vi "GetPktLoss.vi"(8 "error in (no error)":errorcluster, 11 "NetworkPluginNone":refnum<class "NetworkPluginNone.lvclass">) -> (0 "error out":errorcluster, 3 "NetworkPluginNone":refnum<class "NetworkPluginNone.lvclass">)   [LabVIEW 2014, in "NetworkImpairmentPlugins.lvlib" / "NetworkPluginNone.lvclass"]
uses:
  NetworkPluginNone.lvclass
  NetworkImpairmentPluginBase_class/Accessors/Read TimeArray.vi
  NetworkImpairmentPluginBase_class/Accessors/Set PktLoss.vi
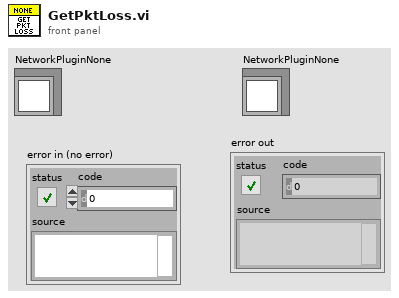
[diagram p1: front panel]
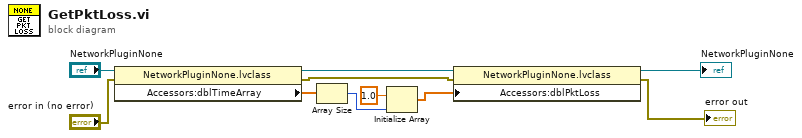
[diagram p0: block diagram]
diagram:
  n1 = property class="NetworkPluginNone.lvclass"(reference="NetworkPluginNone", error in="error in (no error)") -> (reference out=w7:refnum<class "NetworkPluginNone.lvclass">, error out=w1:errorcluster, "Accessors:dblTimeArray"=w9:dbl[])
  n2 = Array Size(array=w9) -> (size(s)=w8:i32)
  n3 = Initialize Array(1.0 ("element"), w8) -> (w5:dbl[])
  n4 = property class="NetworkPluginNone.lvclass"(reference=w7, error in=w1, "Accessors:dblPktLoss"=w5) -> (reference out=→"NetworkPluginNone":refnum<class "NetworkPluginNone.lvclass">, error out=→"error out":errorcluster)
